vi "Global 1.vi"() -> ()   [LabVIEW 2017]
panel:
  out "Station 1 Cycle cmplt":bool
  out "Station 2 Cycle cmplt":bool
  out "PLC Communication STATION 2":bool
  out "PLC Communication STATION 1":bool
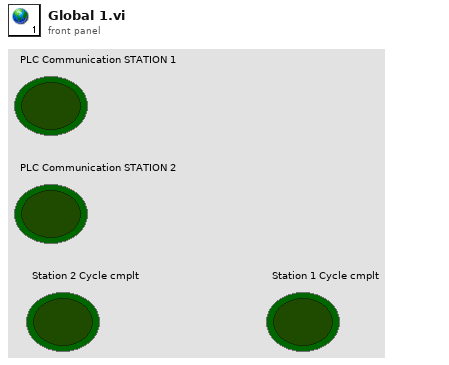
[diagram p1: front panel]
diagram:
